vi "Init OBS.vi"(8 "error in (no error)":errorcluster, 11 "FormulaG App in":refnum<class "FormulaG App.lvclass">) -> (0 "error out":errorcluster, 3 "FormulaG App out":refnum<class "FormulaG App.lvclass">)   [LabVIEW 2024, in "FormulaG.lvlib" / "FormulaG App.lvclass"]
uses:
  FormulaG App.lvclass
  FormulaG App.lvclass/FormulaG App.ctl
  <vilib>/IlluminatedG/IG OBS API/obs-websocket/OBS/OBS.lvclass
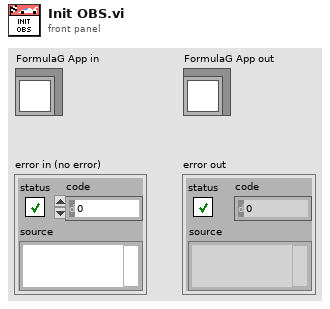
[diagram p1: front panel]
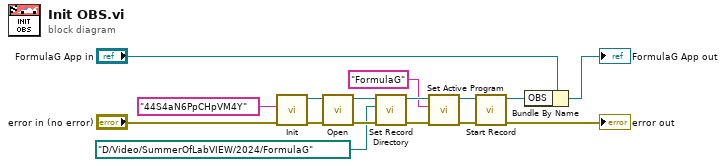
[diagram p0: block diagram]
diagram:
  n1 = call <vilib>:"Init.vi"("error in (no error)"="error in (no error)", "Password (None)"="44S4aN6PpCHpVM4Y") -> ("error out"=w13:errorcluster, "OBS out"=w14:refnum<class "OBS.lvclass">)  [unwired: 8 in]
  n2 = call <vilib>:"Open.vi"("error in (no error)"=w13, "OBS in"=w14) -> ("error out"=w9:errorcluster, "OBS out"=w10:refnum<class "OBS.lvclass">)  [unwired: 8 in]
  n3 = call <vilib>:"Set Record Directory.vi"("error in (no error)"=w9, "Record Directory"=path "D:/Video/SummerOfLabVIEW/2024/FormulaG", "OBS in"=w10) -> ("error out"=w6:errorcluster, "OBS out"=w7:refnum<class "OBS.lvclass">)  [unwired: 7 in]
  n4 = call <vilib>:"Set Active Program.vi"("error in (no error)"=w6, "Scene Name"="FormulaG", "OBS in"=w7) -> ("error out"=w4:errorcluster, "OBS out"=w3:refnum<class "OBS.lvclass">)  [unwired: 7 in]
  n5 = call <vilib>:"Start Record.vi"("error in (no error)"=w4, "OBS in"=w3) -> ("error out"=→"error out":errorcluster, "OBS out"=w2:refnum<class "OBS.lvclass">)  [unwired: 8 in]
  n6 = Bundle By Name(cluster="FormulaG App in", "OBS"=w2) -> (→"FormulaG App out":refnum<class "FormulaG App.lvclass">)
